vi "EPTxBasicExampleRT1.0.vi"() -> ()   [LabVIEW 2022 SP3]
uses:
  <vilib>/rvi/interface/nirviOpenFPGA/nirviOpenFPGA.xnode
  <vilib>/rvi/interface/nirviReadWriteControl/nirviReadWriteControl.xnode
  <vilib>/rvi/interface/Simulation/niFpgaSimulationCallBeginRW.vi
  <vilib>/rvi/errors/niLvFpgaAdjustHostInterfaceError.vi
  <vilib>/Powertrain Controls/Device Drivers/Engine Position Tracking/EPTx/RevA/RT/EPTx - RevA - RT.lvlib
  <vilib>/Platform/TimedLoop/XDataNode/XDataNode.xnode
  <vilib>/Platform/TimedLoop/XDataNode/nitl_modes.ctl
  <vilib>/Platform/TimedLoop/XDataNode/XDNodeRunTimeDep.lvlib
  <vilib>/Platform/TimedLoop/XDataNode/wakeup.ctl
  <vilib>/Platform/TimedLoop/XDataNode/timing_clust.ctl
  <vilib>/rvi/interface/nirviCloseFPGA/nirviCloseFPGA.xnode
  NiFpgaLv.dll
  <vilib>/Utility/error.llb/Error Cluster From Error Code.vi
  <vilib>/Powertrain Controls/Device Drivers/Engine Position Tracking/EPTx/RevA/RT/Controls/Aux Threshold.ctl
  <vilib>/Powertrain Controls/Device Drivers/Engine Position Tracking/EPTx/RevA/RT/Controls/Aux Type.ctl
  <vilib>/Powertrain Controls/Device Drivers/Engine Position Tracking/EPTx/RevA/RT/Controls/Aux Signal.ctl
  <vilib>/Powertrain Controls/Device Drivers/Engine Position Tracking/EPTx/RevA/RT/Controls/Settings - Token.ctl
  <vilib>/Powertrain Controls/Device Drivers/Engine Position Tracking/EPTx/RevA/RT/Controls/Settings - Pattern.ctl
  <vilib>/Powertrain Controls/Device Drivers/Engine Position Tracking/EPTx/RevA/RT/Controls/Direction Detection.ctl
  <vilib>/Powertrain Controls/Device Drivers/Engine Position Tracking/EPTx/RevA/RT/Controls/Settings - Tooth.ctl
  <vilib>/Powertrain Controls/Device Drivers/Engine Position Tracking/EPTx/RevA/RT/Controls/EPTxSettings.ctl
  <vilib>/Powertrain Controls/Device Drivers/Engine Position Tracking/EPTx/RevA/RT/Controls/Pattern.ctl
  <vilib>/Powertrain Controls/Device Drivers/Engine Position Tracking/EPTx/RevA/RT/Controls/EPTxPattern.ctl
  FPGA/EPTx Basic Example FPGA 1.0.vi
  <vilib>/FPGAPlugInAG/Dynamic/niLvFpga_Close_Dynamic.vi
  <vilib>/Powertrain Controls/Device Drivers/Engine Position Tracking/EPTx/RevA/RT/Controls/EPTxState.ctl
  <vilib>/Powertrain Controls/Device Drivers/Engine Position Tracking/EPTx/RevA/RT/Controls/EPTxData.ctl
  <vilib>/Powertrain Controls/Device Drivers/Engine Position Tracking/EPTx/RevA/RT/Controls/EPTxFilters.ctl
  <vilib>/Powertrain Controls/Device Drivers/Engine Position Tracking/EPTx/RevA/FPGA/Controls/EPTxDebug.ctl
  <vilib>/Powertrain Controls/Device Drivers/Engine Position Tracking/EPTx/RevA/FPGA/EPTx - RevA - FPGA.lvlib
  <vilib>/Powertrain Controls/Device Drivers/Engine Position Tracking/EPTx/RevA/RT/Controls/Pattern Config.ctl
  <vilib>/Powertrain Controls/Device Drivers/Engine Position Tracking/EPTx/RevA/RT/Controls/Simulator Config.ctl
  <vilib>/Powertrain Controls/Device Drivers/Engine Position Tracking/EPTx/RevA/RT/Controls/EPTxAAPControl.ctl
  <vilib>/userdefined/High Color/nirio_resource_hc.ctl
  <vilib>/Powertrain Controls/Device Drivers/Engine Position Tracking/EPTx/RevA/FPGA/Controls/EPTxConfig.ctl
  <vilib>/Powertrain Controls/Device Drivers/Engine Position Tracking/EPTx/RevA/FPGA/Controls/EPTxSimulatorConfig.ctl
panel:
  out "EPTxPatternSettings 2":T1
  out "EPTxSettings 2":T3 {"Pattern"."dAngle" format="%#_10g"}
  in  "Injection_DBTDC":sgl=6.0
  in  "Injection_duration[ms]":sgl=2.0
  out "EPTxSimulatorConfig":T11
  out "EPTxConfig":T12
  in  "EPTxPatternSettings":T1={"Rotations"=2, "Cylinders"=6, "Primary"=[{"Angle"=0.0, "State"=FALSE}, {"Angle"=3.0, "State"=TRUE}, {"Angle"=6.0, "State"=FALSE}, {"Angle"=9.0, "State"=TRUE}, {"Angle"=12.0, "State"=FALSE}, {"Angle"=15.0, "State"=TRUE}, {"Angle"=18.0, "State"=FALSE}, {"Angle"=21.0, "State"=TRUE}, {"Angle"=24.0, "State"=FALSE}, {"Angle"=27.0, "State"=TRUE}, {"Angle"=30.0, "State"=FALSE}, {"Angle"=33.0, "State"=TRUE}, {"Angle"=36.0, "State"=FALSE}, {"Angle"=39.0, "State"=TRUE}, {"Angle"=42.0, "State"=FALSE}, {"Angle"=45.0, "State"=TRUE}, {"Angle"=48.0, "State"=FALSE}, {"Angle"=51.0, "State"=TRUE}, {"Angle"=54.0, "State"=FALSE}, {"Angle"=57.0, "State"=TRUE}, {"Angle"=60.0, "State"=FALSE}, {"Angle"=63.0, "State"=TRUE}, {"Angle"=66.0, "State"=FALSE}, {"Angle"=69.0, "State"=TRUE}, {"Angle"=72.0, "State"=FALSE}, {"Angle"=75.0, "State"=TRUE}, {"Angle"=78.0, "State"=FALSE}, {"Angle"=81.0, "State"=TRUE}, {"Angle"=84.0, "State"=FALSE}, {"Angle"=87.0, "State"=TRUE}, {"Angle"=90.0, "State"=FALSE}, {"Angle"=93.0, "State"=TRUE}, {"Angle"=96.0, "State"=FALSE}, {"Angle"=99.0, "State"=TRUE}, {"Angle"=102.0, "State"=FALSE}, {"Angle"=105.0, "State"=TRUE}, {"Angle"=108.0, "State"=FALSE}, {"Angle"=111.0, "State"=TRUE}, {"Angle"=114.0, "State"=FALSE}, {"Angle"=117.0, "State"=TRUE}, {"Angle"=120.0, "State"=FALSE}, {"Angle"=123.0, "State"=TRUE}, {"Angle"=126.0, "State"=FALSE}, {"Angle"=129.0, "State"=TRUE}, {"Angle"=132.0, "State"=FALSE}, {"Angle"=135.0, "State"=TRUE}, {"Angle"=138.0, "State"=FALSE}, {"Angle"=141.0, "State"=TRUE}, {"Angle"=144.0, "State"=FALSE}, {"Angle"=147.0, "State"=TRUE}, {"Angle"=150.0, "State"=FALSE}, {"Angle"=153.0, "State"=TRUE}, {"Angle"=156.0, "State"=FALSE}, {"Angle"=159.0, "State"=TRUE}, {"Angle"=162.0, "State"=FALSE}, {"Angle"=165.0, "State"=TRUE}, {"Angle"=168.0, "State"=FALSE}, {"Angle"=171.0, "State"=TRUE}, {"Angle"=174.0, "State"=FALSE}, {"Angle"=177.0, "State"=TRUE}, {"Angle"=180.0, "State"=FALSE}, {"Angle"=183.0, "State"=TRUE}, {"Angle"=186.0, "State"=FALSE}, {"Angle"=189.0, "State"=TRUE}, {"Angle"=192.0, "State"=FALSE}, {"Angle"=195.0, "State"=TRUE}, {"Angle"=198.0, "State"=FALSE}, {"Angle"=201.0, "State"=TRUE}, {"Angle"=204.0, "State"=FALSE}, {"Angle"=207.0, "State"=TRUE}, {"Angle"=210.0, "State"=FALSE}, {"Angle"=213.0, "State"=TRUE}, {"Angle"=216.0, "State"=FALSE}, {"Angle"=219.0, "State"=TRUE}, {"Angle"=222.0, "State"=FALSE}, {"Angle"=225.0, "State"=TRUE}, {"Angle"=228.0, "State"=FALSE}, {"Angle"=231.0, "State"=TRUE}, {"Angle"=234.0, "State"=FALSE}, {"Angle"=237.0, "State"=TRUE}, {"Angle"=240.0, "State"=FALSE}, {"Angle"=243.0, "State"=TRUE}, {"Angle"=246.0, "State"=FALSE}, {"Angle"=249.0, "State"=TRUE}, {"Angle"=252.0, "State"=FALSE}, {"Angle"=255.0, "State"=TRUE}, {"Angle"=258.0, "State"=FALSE}, {"Angle"=261.0, "State"=TRUE}, {"Angle"=264.0, "State"=FALSE}, {"Angle"=267.0, "State"=TRUE}, {"Angle"=270.0, "State"=FALSE}, {"Angle"=273.0, "State"=TRUE}, {"Angle"=276.0, "State"=FALSE}, {"Angle"=279.0, "State"=TRUE}, {"Angle"=282.0, "State"=FALSE}, {"Angle"=285.0, "State"=TRUE}, {"Angle"=288.0, "State"=FALSE}, {"Angle"=291.0, "State"=TRUE}, {"Angle"=294.0, "State"=FALSE}, {"Angle"=297.0, "State"=TRUE}, {"Angle"=300.0, "State"=FALSE}, {"Angle"=303.0, "State"=TRUE}, {"Angle"=306.0, "State"=FALSE}, {"Angle"=309.0, "State"=TRUE}, {"Angle"=312.0, "State"=FALSE}, {"Angle"=315.0, "State"=TRUE}, {"Angle"=318.0, "State"=FALSE}, {"Angle"=321.0, "State"=TRUE}, {"Angle"=324.0, "State"=FALSE}, {"Angle"=327.0, "State"=TRUE}, {"Angle"=330.0, "State"=FALSE}, {"Angle"=333.0, "State"=TRUE}, {"Angle"=336.0, "State"=FALSE}, {"Angle"=339.0, "State"=TRUE}, {"Angle"=342.0, "State"=FALSE}, {"Angle"=345.0, "State"=TRUE}, {"Angle"=360.0, "State"=FALSE}, {"Angle"=363.0, "State"=TRUE}, {"Angle"=366.0, "State"=FALSE}, {"Angle"=369.0, "State"=TRUE}, {"Angle"=372.0, "State"=FALSE}, {"Angle"=375.0, "State"=TRUE}, {"Angle"=378.0, "State"=FALSE}, {"Angle"=381.0, "State"=TRUE}, {"Angle"=384.0, "State"=FALSE}, {"Angle"=387.0, "State"=TRUE}, {"Angle"=390.0, "State"=FALSE}, {"Angle"=393.0, "State"=TRUE}, {"Angle"=396.0, "State"=FALSE}, {"Angle"=399.0, "State"=TRUE}, {"Angle"=402.0, "State"=FALSE}, {"Angle"=405.0, "State"=TRUE}, {"Angle"=408.0, "State"=FALSE}, {"Angle"=411.0, "State"=TRUE}, {"Angle"=414.0, "State"=FALSE}, {"Angle"=417.0, "State"=TRUE}, {"Angle"=420.0, "State"=FALSE}, {"Angle"=423.0, "State"=TRUE}, {"Angle"=426.0, "State"=FALSE}, {"Angle"=429.0, "State"=TRUE}, {"Angle"=432.0, "State"=FALSE}, {"Angle"=435.0, "State"=TRUE}, {"Angle"=438.0, "State"=FALSE}, {"Angle"=441.0, "State"=TRUE}, {"Angle"=444.0, "State"=FALSE}, {"Angle"=447.0, "State"=TRUE}, {"Angle"=450.0, "State"=FALSE}, {"Angle"=453.0, "State"=TRUE}, {"Angle"=456.0, "State"=FALSE}, {"Angle"=459.0, "State"=TRUE}, {"Angle"=462.0, "State"=FALSE}, {"Angle"=465.0, "State"=TRUE}, {"Angle"=468.0, "State"=FALSE}, {"Angle"=471.0, "State"=TRUE}, {"Angle"=474.0, "State"=FALSE}, {"Angle"=477.0, "State"=TRUE}, {"Angle"=480.0, "State"=FALSE}, {"Angle"=483.0, "State"=TRUE}, {"Angle"=486.0, "State"=FALSE}, {"Angle"=489.0, "State"=TRUE}, {"Angle"=492.0, "State"=FALSE}, {"Angle"=495.0, "State"=TRUE}, {"Angle"=498.0, "State"=FALSE}, {"Angle"=501.0, "State"=TRUE}, {"Angle"=504.0, "State"=FALSE}, {"Angle"=507.0, "State"=TRUE}, {"Angle"=510.0, "State"=FALSE}, {"Angle"=513.0, "State"=TRUE}, {"Angle"=516.0, "State"=FALSE}, {"Angle"=519.0, "State"=TRUE}, {"Angle"=522.0, "State"=FALSE}, {"Angle"=525.0, "State"=TRUE}, {"Angle"=528.0, "State"=FALSE}, {"Angle"=531.0, "State"=TRUE}, {"Angle"=534.0, "State"=FALSE}, {"Angle"=537.0, "State"=TRUE}, {"Angle"=540.0, "State"=FALSE}, {"Angle"=543.0, "State"=TRUE}, {"Angle"=546.0, "State"=FALSE}, {"Angle"=549.0, "State"=TRUE}, {"Angle"=552.0, "State"=FALSE}, {"Angle"=555.0, "State"=TRUE}, {"Angle"=558.0, "State"=FALSE}, {"Angle"=561.0, "State"=TRUE}, {"Angle"=564.0, "State"=FALSE}, {"Angle"=567.0, "State"=TRUE}, {"Angle"=570.0, "State"=FALSE}, {"Angle"=573.0, "State"=TRUE}, {"Angle"=576.0, "State"=FALSE}, {"Angle"=579.0, "State"=TRUE}, {"Angle"=582.0, "State"=FALSE}, {"Angle"=585.0, "State"=TRUE}, {"Angle"=588.0, "State"=FALSE}, {"Angle"=591.0, "State"=TRUE}, {"Angle"=594.0, "State"=FALSE}, {"Angle"=597.0, "State"=TRUE}, {"Angle"=600.0, "State"=FALSE}, {"Angle"=603.0, "State"=TRUE}, {"Angle"=606.0, "State"=FALSE}, {"Angle"=609.0, "State"=TRUE}, {"Angle"=612.0, "State"=FALSE}, {"Angle"=615.0, "State"=TRUE}, {"Angle"=618.0, "State"=FALSE}, {"Angle"=621.0, "State"=TRUE}, {"Angle"=624.0, "State"=FALSE}, {"Angle"=627.0, "State"=TRUE}, {"Angle"=630.0, "State"=FALSE}, {"Angle"=633.0, "State"=TRUE}, {"Angle"=636.0, "State"=FALSE}, {"Angle"=639.0, "State"=TRUE}, {"Angle"=642.0, "State"=FALSE}, {"Angle"=645.0, "State"=TRUE}, {"Angle"=648.0, "State"=FALSE}, {"Angle"=651.0, "State"=TRUE}, {"Angle"=654.0, "State"=FALSE}, {"Angle"=657.0, "State"=TRUE}, {"Angle"=660.0, "State"=FALSE}, {"Angle"=663.0, "State"=TRUE}, {"Angle"=666.0, "State"=FALSE}, {"Angle"=669.0, "State"=TRUE}, {"Angle"=672.0, "State"=FALSE}, {"Angle"=675.0, "State"=TRUE}, {"Angle"=678.0, "State"=FALSE}, {"Angle"=681.0, "State"=TRUE}, {"Angle"=684.0, "State"=FALSE}, {"Angle"=687.0, "State"=TRUE}, {"Angle"=690.0, "State"=FALSE}, {"Angle"=693.0, "State"=TRUE}, {"Angle"=696.0, "State"=FALSE}, {"Angle"=699.0, "State"=TRUE}, {"Angle"=702.0, "State"=FALSE}, {"Angle"=705.0, "State"=TRUE}], "Aux 1"=[{"Angle"=12.0, "State"=TRUE}, {"Angle"=24.0, "State"=FALSE}, {"Angle"=48.0, "State"=TRUE}, {"Angle"=60.0, "State"=FALSE}, {"Angle"=132.0, "State"=TRUE}, {"Angle"=144.0, "State"=FALSE}, {"Angle"=198.0, "State"=TRUE}, {"Angle"=252.0, "State"=TRUE}, {"Angle"=264.0, "State"=FALSE}, {"Angle"=318.0, "State"=TRUE}, {"Angle"=372.0, "State"=TRUE}, {"Angle"=384.0, "State"=FALSE}, {"Angle"=438.0, "State"=TRUE}, {"Angle"=492.0, "State"=TRUE}, {"Angle"=504.0, "State"=FALSE}, {"Angle"=558.0, "State"=TRUE}, {"Angle"=612.0, "State"=TRUE}, {"Angle"=624.0, "State"=FALSE}, {"Angle"=678.0, "State"=TRUE}], "Aux 2"=[{"Angle"=12.0, "State"=TRUE}, {"Angle"=24.0, "State"=FALSE}, {"Angle"=48.0, "State"=TRUE}, {"Angle"=60.0, "State"=FALSE}, {"Angle"=132.0, "State"=TRUE}, {"Angle"=144.0, "State"=FALSE}, {"Angle"=198.0, "State"=TRUE}, {"Angle"=252.0, "State"=TRUE}, {"Angle"=264.0, "State"=FALSE}, {"Angle"=318.0, "State"=TRUE}, {"Angle"=372.0, "State"=TRUE}, {"Angle"=384.0, "State"=FALSE}, {"Angle"=438.0, "State"=TRUE}, {"Angle"=492.0, "State"=TRUE}, {"Angle"=504.0, "State"=FALSE}, {"Angle"=558.0, "State"=TRUE}, {"Angle"=612.0, "State"=TRUE}, {"Angle"=624.0, "State"=FALSE}, {"Angle"=678.0, "State"=TRUE}], "Aux 3"=[], "Aux 4"=[]}
  in  "load_备用":bool
  out "EPTxSettings":T3 {"Pattern"."dAngle" format="%#_10g"}
  in  "EPTxAAPControl_6str":T13={"Enable"=FALSE, "Rising [DBTDC]"=12.0, "Falling [DBTDC]"=-12.0}
  in  "EPTxAAPControl_5str":T13={"Enable"=FALSE, "Rising [DBTDC]"=12.0, "Falling [DBTDC]"=-12.0}
  in  "EPTxAAPControl_4str":T13={"Enable"=FALSE, "Rising [DBTDC]"=12.0, "Falling [DBTDC]"=-12.0}
  in  "EPTxAAPControl_3str":T13={"Enable"=FALSE, "Rising [DBTDC]"=12.0, "Falling [DBTDC]"=-12.0}
  in  "EPTxAAPControl_2str":T13={"Enable"=FALSE, "Rising [DBTDC]"=12.0, "Falling [DBTDC]"=-12.0}
  out "Loop":u32
  in  "资源名称":T14="PXI1Slot7" caption="RIO设备"
  out "Config Loading":bool
  in  "EPTxAAPControl_1str":T13={"Enable"=FALSE, "Rising [DBTDC]"=12.0, "Falling [DBTDC]"=-12.0}
  out "Pattern Loading":bool
  in  "SimulatorConfig":T15={"Sim Speed [RPM]"=1000.0, "Ramp Rate [RPM/s]"=50.0, "Rotations"=2, "Pause"=FALSE, "Pause Angle [CAD]"=0.0, "Max Offset [RPM]"=0.0, "Cylinders"=6}
  out "Sim Loading":bool
  in  "PatternConfig":T16 {"Max Rate [Hz]" format="%#_3p"}
  out "error out":errorcluster
  out "RT Loop Iteration Duration":i64 caption="[ms]"
  out "EPTxDebug":T17={"Sync"=TRUE, "CycleCount"=146.0, "StartCAD"=0.0, "EndCAD"=123.3046875}
  in  "History [CAD]":u8=63
  in  "EPTxFilters":T18={"Primary [s]"=5e-06, "Aux 1 [s]"=5e-06, "Aux 2 [s]"=0.0, "Aux 3 [s]"=0.0, "Aux 4 [s]"=0.0} {"Aux 4 [s]" format="%#_6p"; "Aux 3 [s]" format="%#_6p"; "Aux 2 [s]" format="%#_6p"; "Aux 1 [s]" format="%#_6p"; "Primary [s]" format="%#_6p"}
  in  "Stall Speed [RPM]":sgl=200.0
  in  "Configuration Filename":string="YC-6kcfg.EPTx"
  in  "Pattern Filename":string="YC-6kcfg.EPTxP"
  in  "Load":bool
  out "EPTxData":T19={"Sync"=TRUE, "CurrentCAD"=122.91406, "Speed [RPM]"=999.75, "Config"=FALSE, "Rcvg Primary"=TRUE, "Stall"=FALSE, "Overflow"=FALSE, "Ratio Error"=FALSE, "Pattern Error"=FALSE, "Aux Warning"=FALSE, "Watchdog Error"=FALSE}
  in  "EPTxState":T20={"Sync Enable"=TRUE, "Clear Errors"=FALSE, "Sim Enable"=FALSE, "Sim Speed [RPM]"=1000.0}
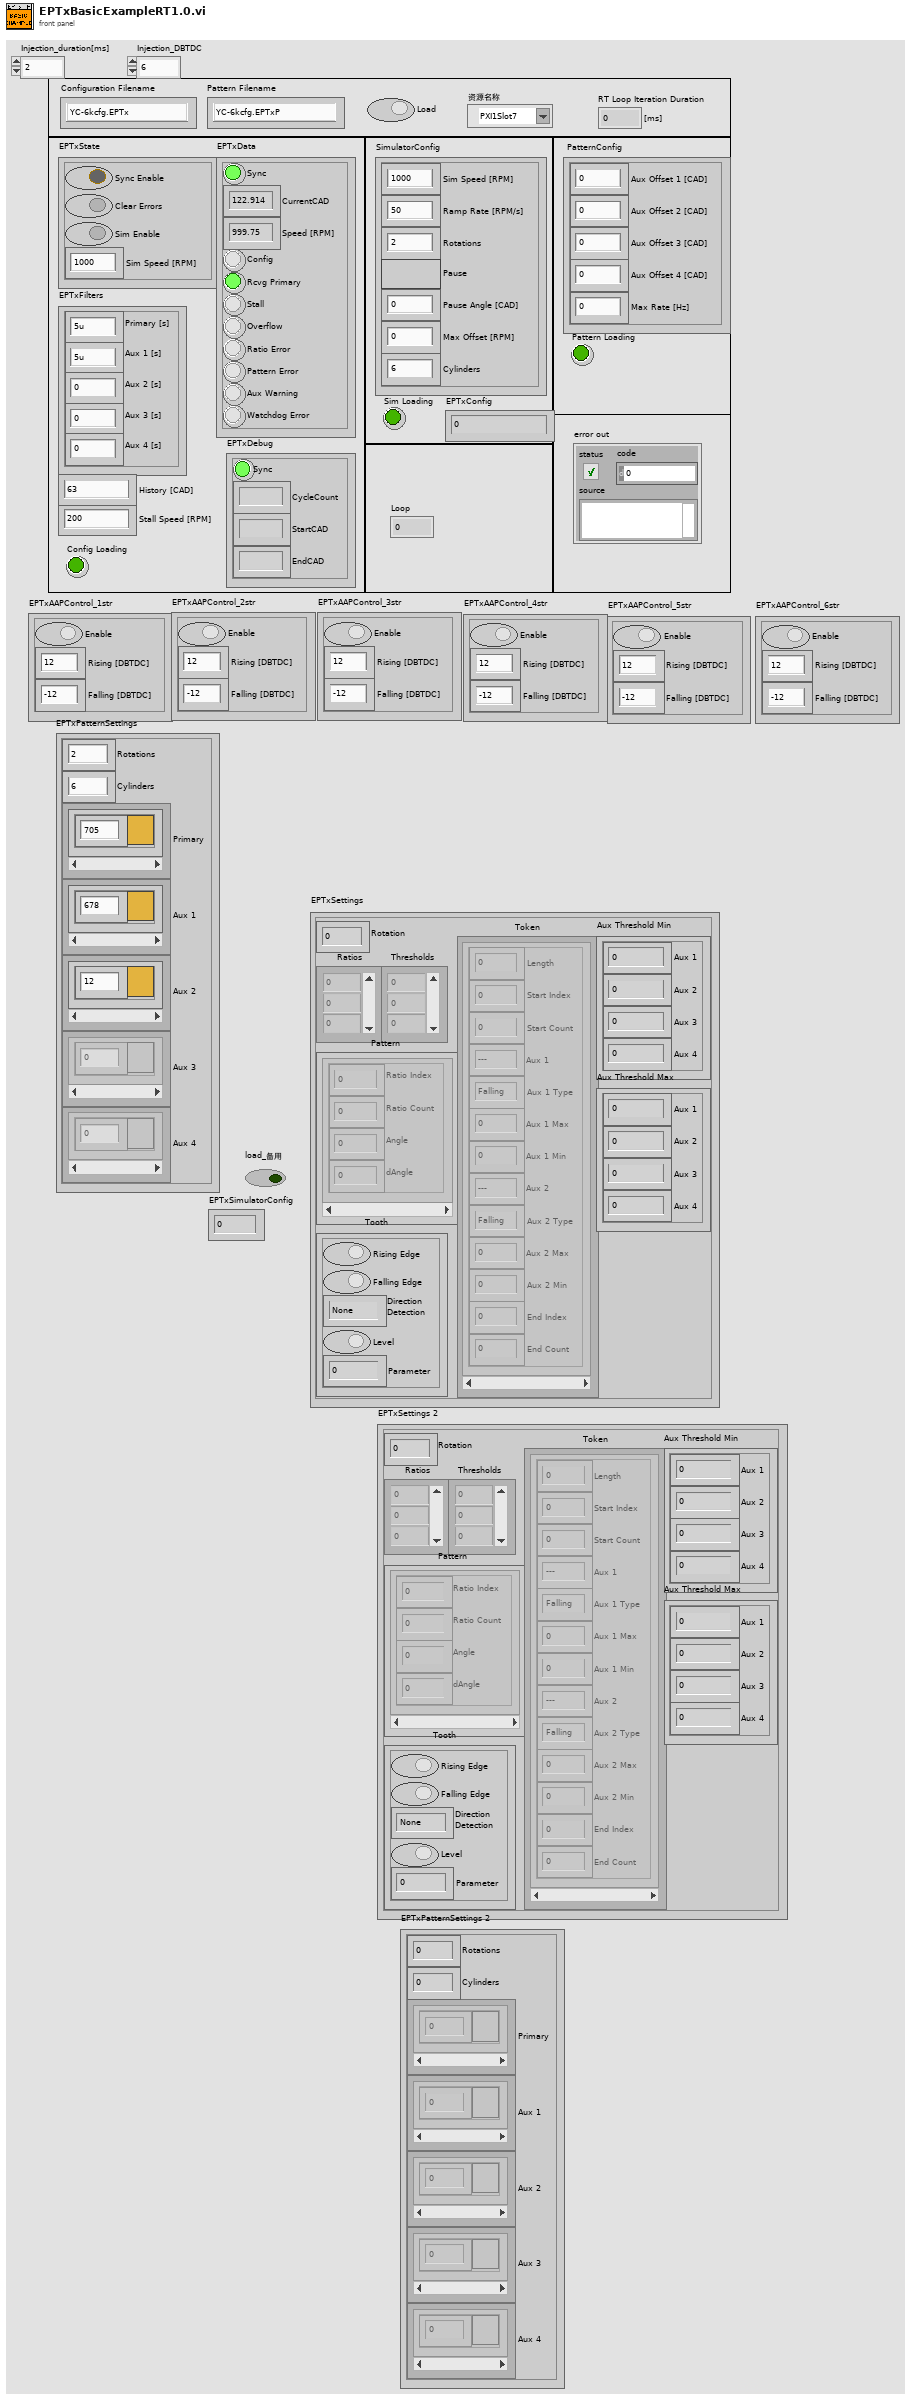
[diagram p1: front panel]
types:
  T1 = typedef "EPTx - RevA - RT.lvlib/EPTxPattern.ctl" = cluster{"Rotations":u8, "Cylinders":u8, "Primary":T2[], "Aux 1":T2[], "Aux 2":T2[], "Aux 3":T2[], "Aux 4":T2[]}
  T2 = typedef "EPTx - RevA - RT.lvlib/Pattern.ctl" = cluster{"Angle":sgl, "State":bool}
  T3 = typedef "EPTx - RevA - RT.lvlib/EPTxSettings.ctl" = cluster{"Rotation":u8, "Ratios":sgl[], "Thresholds":sgl[], "Tooth":T4, "Pattern":T6[], "Token":T7[], "Aux Threshold Min":T10, "Aux Threshold Max":T10}
  T4 = typedef "EPTx - RevA - RT.lvlib/Settings - Tooth.ctl" = cluster{"Rising Edge":bool, "Falling Edge":bool, "Direction\nDetection":T5, "Level":bool, "Parameter":sgl}
  T5 = typedef "EPTx - RevA - RT.lvlib/Direction Detection.ctl" = enum16{"None", "Aux Signal", "Length"}
  T6 = typedef "EPTx - RevA - RT.lvlib/Settings - Pattern.ctl" = cluster{"Ratio Index":u8, "Ratio Count":u16, "Angle":sgl, "dAngle":sgl}
  T7 = typedef "EPTx - RevA - RT.lvlib/Settings - Token.ctl" = cluster{"Length":u16, "Start Index":u8, "Start Count":u16, "Aux 1":T8, "Aux 1 Type":T9, "Aux 1 Max":u16, "Aux 1 Min":u16, "Aux 2":T8, "Aux 2 Type":T9, "Aux 2 Max":u16, "Aux 2 Min":u16, "End Index":u8, "End Count":u16}
  T8 = typedef "EPTx - RevA - RT.lvlib/Aux Signal.ctl" = enum8{"---", "Aux 1", "Aux 2", "Aux 3", "Aux 4"}
  T9 = typedef "EPTx - RevA - RT.lvlib/Aux Type.ctl" = enum8{"Falling", "Rising", "Low", "High", "Ratio"}
  T10 = typedef "EPTx - RevA - RT.lvlib/Aux Threshold.ctl" = cluster{"Aux 1":sgl, "Aux 2":sgl, "Aux 3":sgl, "Aux 4":sgl}
  T11 = typedef "EPTx - RevA - FPGA.lvlib/EPTxSimulatorConfig.ctl" = u32
  T12 = typedef "EPTx - RevA - FPGA.lvlib/EPTxConfig.ctl" = u64
  T13 = typedef "EPTx - RevA - RT.lvlib/EPTxAAPControl.ctl" = cluster{"Enable":bool, "Rising [DBTDC]":sgl, "Falling [DBTDC]":sgl}
  T14 = typedef "nirio_resource_hc.ctl" = tag
  T15 = typedef "EPTx - RevA - RT.lvlib/Simulator Config.ctl" = cluster{"Sim Speed [RPM]":sgl, "Ramp Rate [RPM/s]":sgl, "Rotations":u8, "Pause":bool, "Pause Angle [CAD]":sgl, "Max Offset [RPM]":sgl, "Cylinders":u8}
  T16 = typedef "EPTx - RevA - RT.lvlib/Pattern Config.ctl" = cluster{"Aux Offset 1 [CAD]":sgl, "Aux Offset 2 [CAD]":sgl, "Aux Offset 3 [CAD]":sgl, "Aux Offset 4 [CAD]":sgl, "Max Rate [Hz]":sgl}
  T17 = typedef "EPTx - RevA - FPGA.lvlib/EPTxDebug.ctl" = cluster{"Sync":bool, "CycleCount":fxp<+,8,8>, "StartCAD":fxp<+,18,11>, "EndCAD":fxp<+,18,11>}
  T18 = typedef "EPTx - RevA - RT.lvlib/EPTxFilters.ctl" = cluster{"Primary [s]":sgl, "Aux 1 [s]":sgl, "Aux 2 [s]":sgl, "Aux 3 [s]":sgl, "Aux 4 [s]":sgl}
  T19 = typedef "EPTx - RevA - RT.lvlib/EPTxData.ctl" = cluster{"Sync":bool, "CurrentCAD":sgl, "Speed [RPM]":sgl, "Config":bool, "Rcvg Primary":bool, "Stall":bool, "Overflow":bool, "Ratio Error":bool, "Pattern Error":bool, "Aux Warning":bool, "Watchdog Error":bool}
  T20 = typedef "EPTx - RevA - RT.lvlib/EPTxState.ctl" = cluster{"Sync Enable":bool, "Clear Errors":bool, "Sim Enable":bool, "Sim Speed [RPM]":sgl}
  T21 = typedef "XDNodeRunTimeDep.lvlib/timing_clust.ctl" = cluster{"Expected End [f-1]":u64, "Actual End [f-1]":u64, "Finished Late? [f-1]":bool, "Expected End [i-1]":u64, "Actual End [i-1]":u64, "Finished Late? [i-1]":bool, "Expected Start [i]":u64, "Actual Start [i]":u64, "Expected Start [f]":u64, "Actual Start [f]":u64, "Source Name":string, "Structure Name":string, "Period":i64, "Deadline":i64, "Offset":i64, "Start":i64, "Priority":i32, "Timeout":i32, "Mode":T22, "Wakeup Reason":T23, "Error":errorcluster, "Source Type":string, "Secondary Source Type":string, "Global End Time":u64, "Global Start Time":u64, "Frame Duration":u64, "Iteration Duration":u64, "Assigned CPU":i32, "I/O Scan Engine Mode":u32}
  T22 = typedef "XDNodeRunTimeDep.lvlib/nitl_modes.ctl" = enum32{"No Change", "Process missed periods, maintain original phase", "Discard missed periods, maintain original phase", "Process missed periods, ignore original phase", "Discard missed periods, ignore original phase"}
  T23 = typedef "XDNodeRunTimeDep.lvlib/wakeup.ctl" = enum32{"Normal", "Aborted", "Asynchronous wakeup", "Timing source error", "Timed loop error", "Timeout"}
  T24 = cluster{"Cylinder6_H_R [CAD]":fxp<+,18,11>, "Cylinder6_H_F [CAD]":fxp<+,18,11>}
  T25 = cluster{"Cylinder5_H_R [CAD]":fxp<+,18,11>, "Cylinder5_H_F [CAD]":fxp<+,18,11>}
  T26 = cluster{"Cylinder4_H_R [CAD]":fxp<+,18,11>, "Cylinder4_H_F [CAD]":fxp<+,18,11>}
  T27 = cluster{"Cylinder3_H_R [CAD]":fxp<+,18,11>, "Cylinder3_H_F [CAD]":fxp<+,18,11>}
  T28 = cluster{"Cylinder2_H_R [CAD]":fxp<+,18,11>, "Cylinder2_H_F [CAD]":fxp<+,18,11>}
  T29 = cluster{"Cylinder1_H_R [CAD]":fxp<+,18,11>, "Cylinder1_H_F [CAD]":fxp<+,18,11>}
  T30 = cluster{"Sync":bool, "CurrentCAD":fxp<+,18,11>, "MaxCAD":fxp<+,11,11>, "HistoryCAD":fxp<+,11,11>, "CADRate":fxp<+,22,8>, "AvgSpeed":fxp<+,17,15>, "Config":bool, "Rcvg Primary":bool, "Stall":bool, "Overflow":bool, "Ratio Error":bool, "Pattern Error":bool, "Aux Warning":bool, "Watchdog Error":bool}
  T31 = typedef "EPTx - RevA - FPGA.lvlib/EPTxControl.ctl" = cluster{"Sync Enable":bool, "Clear Errors":bool, "Sim Enable":bool, "Sim Rate":fxp<+,24,6>, "Watchdog":bool}
  T32 = typedef "EPTx - RevA - FPGA.lvlib/EPTxPatternConfig.ctl" = cluster{"Address":fxp<+,14,14>, "Pattern":T33}
  T33 = typedef "EPTx - RevA - FPGA.lvlib/Patterns.ctl" = cluster{"Primary":fxp<+,19,12>, "Primary State":bool, "Aux 1":fxp<+,19,12>, "Aux 1 State":bool, "Aux 2":fxp<+,19,12>, "Aux 2 State":bool, "Aux 3":fxp<+,19,12>, "Aux 3 State":bool, "Aux 4":fxp<+,19,12>, "Aux 4 State":bool}
  T34 = cluster{"Sync":bool, "CycleCount":fxp<+,8,8>, "StartCAD":fxp<+,18,11>, "EndCAD":fxp<+,18,11>}
  T35 = typedef "EPTx - RevA - FPGA.lvlib/EPTxAAPControl.ctl" = cluster{"Enable":bool, "RisingCAD":fxp<+,18,11>, "FallingCAD":fxp<+,18,11>}
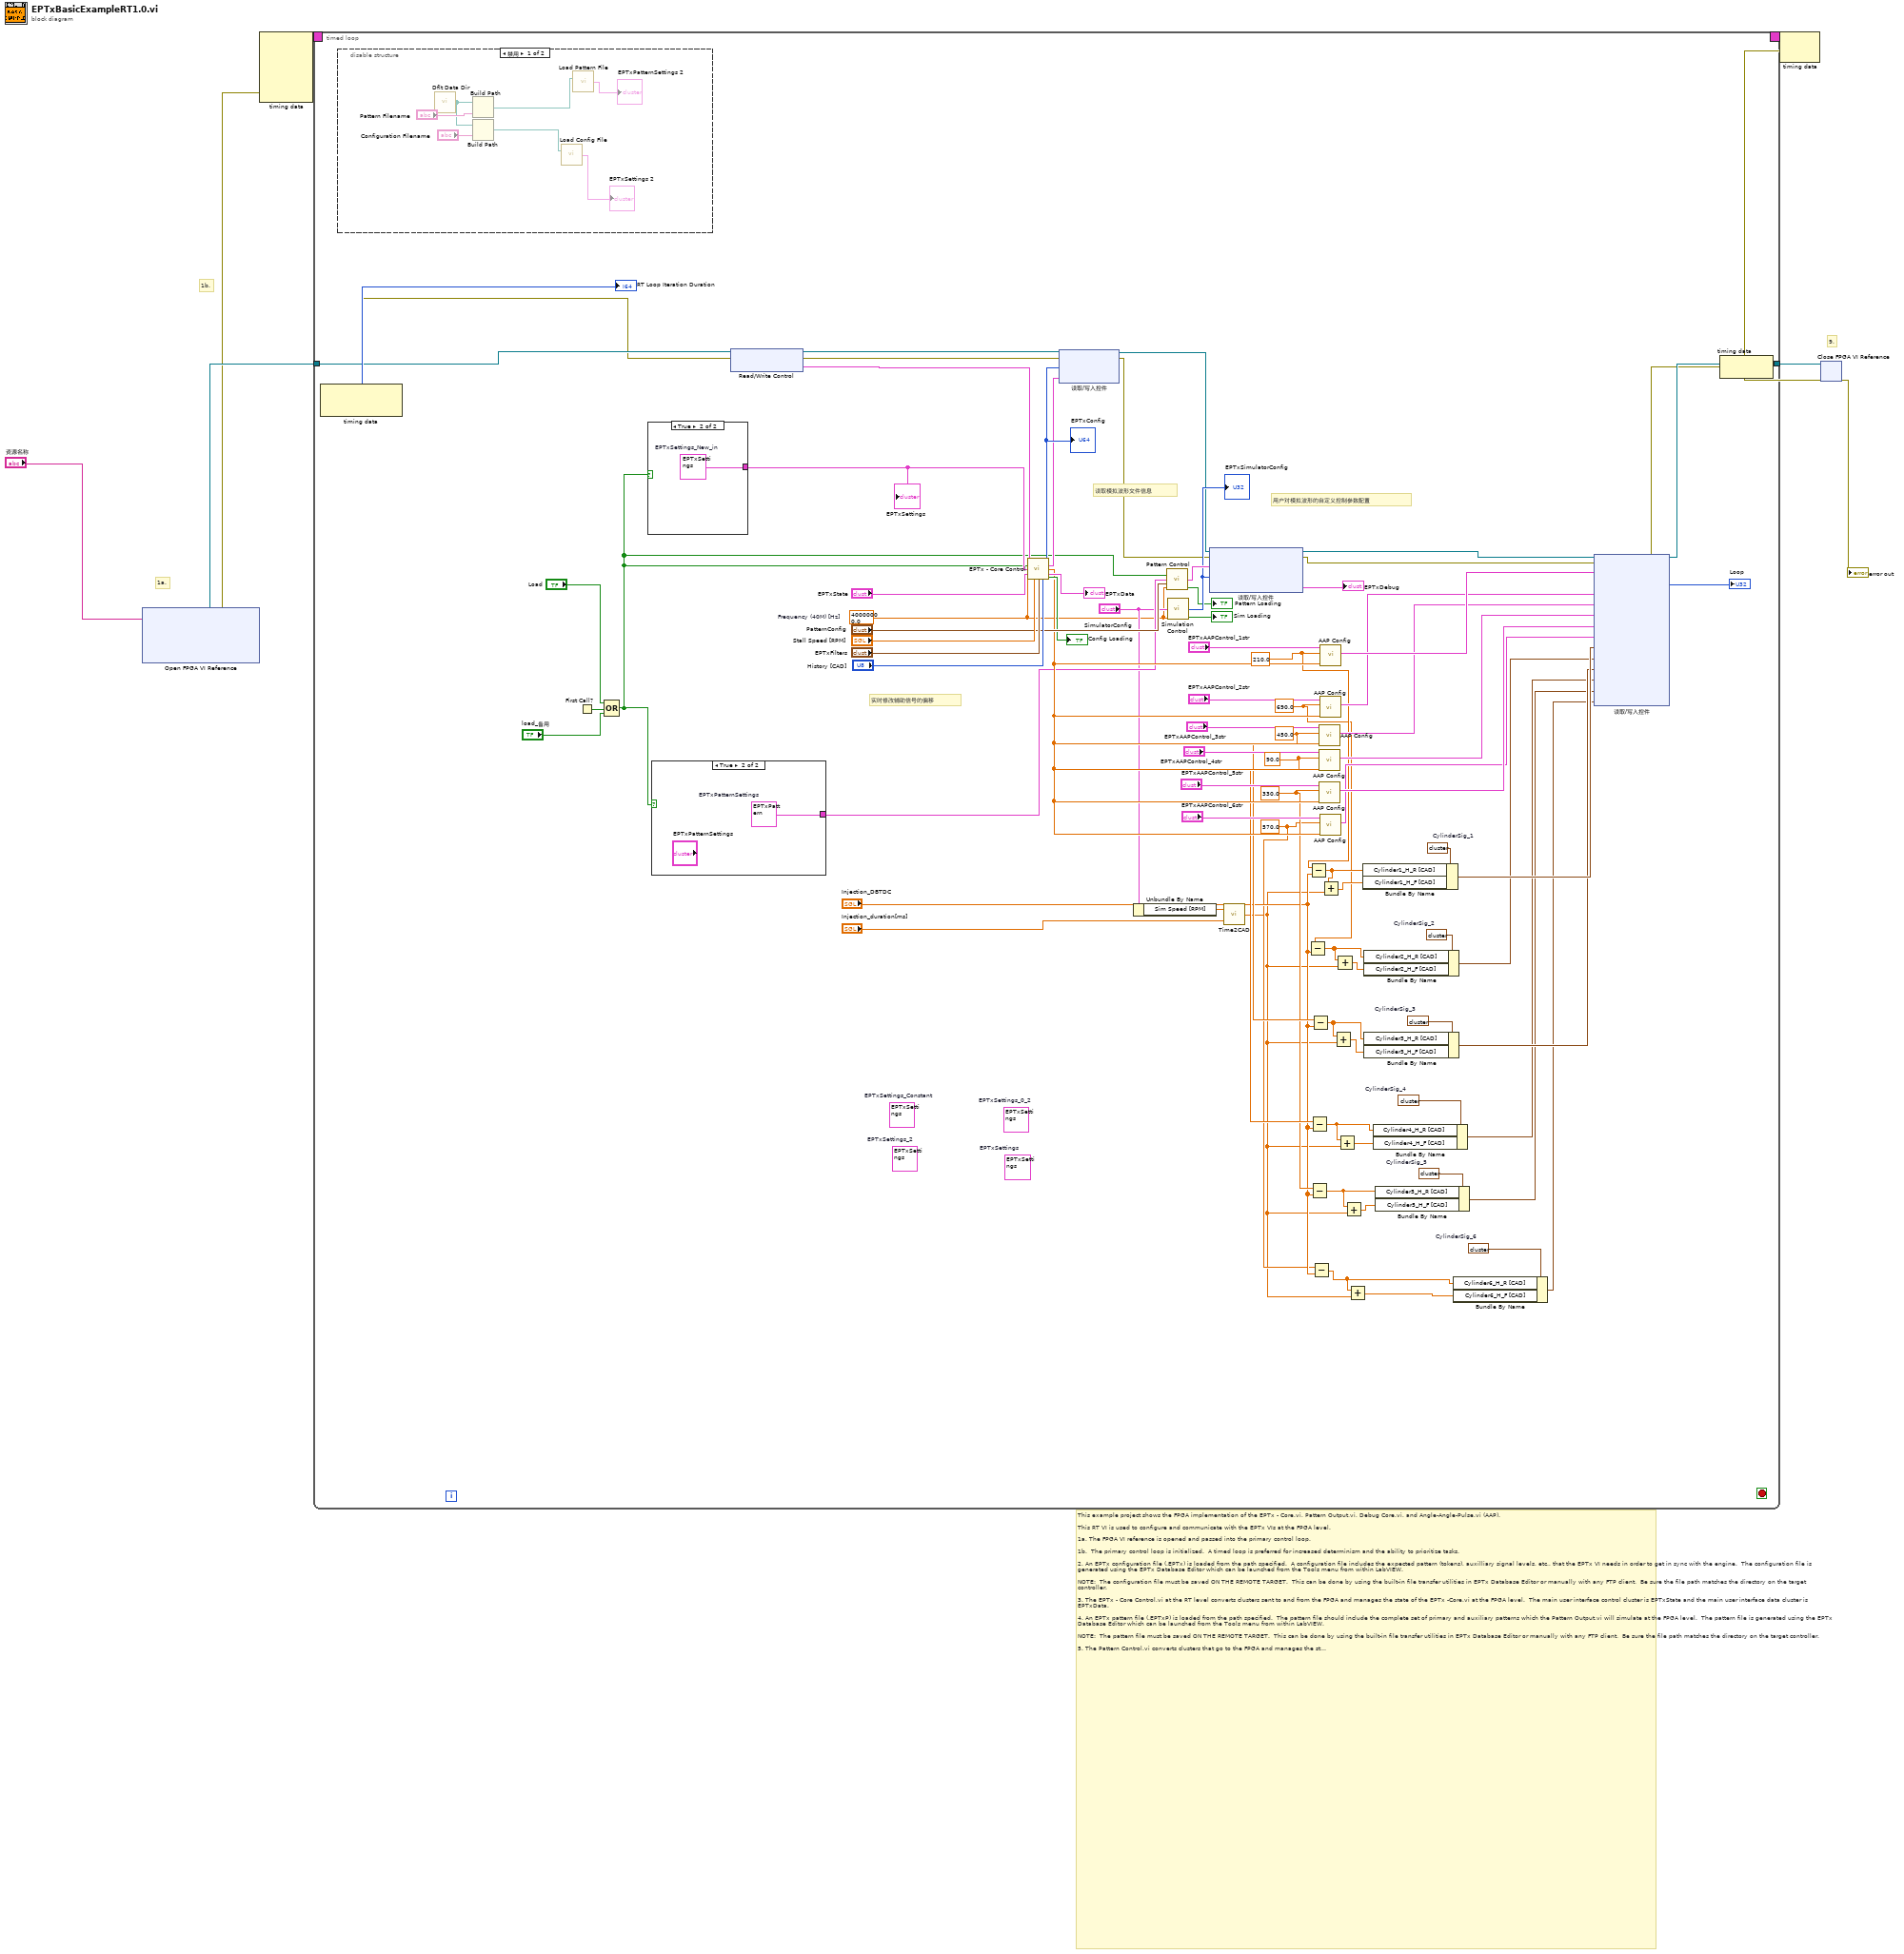
[diagram p0: block diagram]
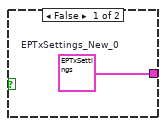
[diagram p3: hidden frame]
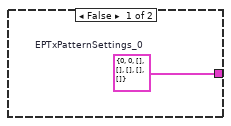
[diagram p4: hidden frame]
diagram:
  # "9."
  # "1b."
  # "1a."
  # "This example project shows the FPGA implementation of the EPTx - Core.vi, Pattern Output.vi, Debug Core.vi, and Angle-Angle-Pulse.vi (AAP).\n\nThis RT VI is used to configure and communicate with the EPTx VIs at the FPGA level.\n\n1a. The FPGA VI reference is opened and passed into the primary control loop.\n\n1b.  The primary control loop is initialized.  A timed loop is preferred for increased determinism and the ability to prioritize tasks.\n\n2. An EPTx configuration file (.EPTx) is loaded from the path specified.  A configuration file includes the expected pattern (tokens), auxilliary signal levels, etc., that the EPTx VI needs in order to get in sync with the engine.  The configuration file is generated using the EPTx Database Editor which can be launched from the Tools menu from within LabVIEW.\n\nNOTE:  The configuration file must be saved ON THE REMOTE TARGET.  This can be done by using the built-in file transfer utilities in EPTx Database Editor or manually with any FTP client.  Be sure the file path matches the directory on the target controller.\n\n3. The EPTx - Core Control.vi at the RT level converts clusters sent to and from the FPGA and manages the state of the EPTx -Core.vi at the FPGA level.  The main user interface control cluster is EPTxState and the main user interface data cluster is EPTxData.\n\n4. An EPTx pattern file (.EPTxP) is loaded from the path specified.  The pattern file should include the complete set of primary and auxiliary patterns which the Pattern Output.vi will simulate at the FPGA level.  The pattern file is generated using the EPTx Database Editor which can be launched from the Tools menu from within LabVIEW.\n\nNOTE:  The pattern file must be saved ON THE REMOTE TARGET.  This can be done by using the built-in file transfer utilities in EPTx Database Editor or manually with any FTP client.  Be sure the file path matches the directory on the target controller.\n\n5. The Pattern Control.vi converts clusters that go to the FPGA and manages the state of the Pattern Output.vi at the FPGA level.  The main user interface control cluster is Pattern Config.  The 'Loading' output indicates the RT VI is busy sending information to the FPGA.\n\n6.  The Simulation Control.vi converts clusters that go to the FPGA and manages the state of the Simulator.vi at the FPGA level.  The main user interface control cluster is Simulator Config.  The 'Loading' output indicates the RT VI is busy sending information to the FPGA.\n\n7. The EPTxDebug cluster reports data from the Debug Core.vi at the FPGA level which includes information that may help the user debug issues with achieving or losing sync.\n\n8. Controls to EPTx Extra blocks.  In this example, an Angle-Angle-Pulse (AAP) VI is used to generate an engine-synchronous boolean pulse.\n\n9. Close the FPGA VI reference."
  n1 = xnode "Open FPGA VI Reference"("resource name"="资源名称") -> ("FPGA VI Reference Out"=w8:refnum<k20>, "error out"=w3:errorcluster)  [unwired: 1 in]
  n2 = node-c288(w3) -> (w7:T21)  [unwired: 4 in]
  n3 = timed-loop {
    tunnel: w8 -> [w53]
    timing: w7 -> [_]
    timing-out: [_] -> w6
    tunnel: [w80] -> w5
    stop <- _ stop-if-true
    w16 = T24 {"Cylinder6_H_R [CAD]"=0.0, "Cylinder6_H_F [CAD]"=0.0}  # CylinderSig_6
    w24 = T25 {"Cylinder5_H_R [CAD]"=324.0, "Cylinder5_H_F [CAD]"=330.0}  # CylinderSig_5
    w29 = T26 {"Cylinder4_H_R [CAD]"=90.0, "Cylinder4_H_F [CAD]"=100.0}  # CylinderSig_4
    w35 = T27 {"Cylinder3_H_R [CAD]"=444.0, "Cylinder3_H_F [CAD]"=450.0}  # CylinderSig_3
    w38 = T28 {"Cylinder2_H_R [CAD]"=684.0, "Cylinder2_H_F [CAD]"=690.0}  # CylinderSig_2
    w42 = T29 {"Cylinder1_H_R [CAD]"=204.0, "Cylinder1_H_F [CAD]"=210.0}  # CylinderSig_1
    (unwired) T3 {"Rotation"=2, "Ratios"=[0.33333334, 1.0, 3.0], "Thresholds"=[0.16666667, 0.6666667, 0.6666667, 2.0, 2.0, 4.0, 999.0], "Tooth"={"Rising Edge"=TRUE, "Falling Edge"=FALSE, "Direction\nDetection"=enum."None", "Level"=FALSE, "Parameter"=0.0}, "Pattern"=[{"Ratio Index"=0, "Ratio Count"=1, "Angle"=0.0, "dAngle"=6.0}, {"Ratio Index"=1, "Ratio Count"=56, "Angle"=6.0, "dAngle"=6.0}, {"Ratio Index"=2, "Ratio Count"=1, "Angle"=342.0, "dAngle"=18.0}, {"Ratio Index"=0, "Ratio Count"=1, "Angle"=360.0, "dAngle"=6.0}, {"Ratio Index"=1, "Ratio Count"=56, "Angle"=366.0, "dAngle"=6.0}, {"Ratio Index"=2, "Ratio Count"=1, "Angle"=702.0, "dAngle"=18.0}], "Token"=[{"Length"=1, "Start Index"=5, "Start Count"=0, "Aux 1"=enum."---", "Aux 1 Type"=enum."Falling", "Aux 1 Max"=0, "Aux 1 Min"=0, "Aux 2"=enum."Aux 2", "Aux 2 Type"=enum."Ratio", "Aux 2 Max"=73, "Aux 2 Min"=73, "End Index"=0, "End Count"=0}], "Aux Threshold Min"={"Aux 1"=2.3333333, "Aux 2"=1.4285715, "Aux 3"=0.0, "Aux 4"=0.0}, "Aux Threshold Max"={"Aux 1"=2.3333333, "Aux 2"=1.4285715, "Aux 3"=999.0, "Aux 4"=999.0}}  # EPTxSettings
    (unwired) T3 {"Rotation"=0, "Ratios"=[], "Thresholds"=[], "Tooth"={"Rising Edge"=FALSE, "Falling Edge"=FALSE, "Direction\nDetection"=enum."None", "Level"=FALSE, "Parameter"=0.0}, "Pattern"=[], "Token"=[], "Aux Threshold Min"={"Aux 1"=0.0, "Aux 2"=0.0, "Aux 3"=0.0, "Aux 4"=0.0}, "Aux Threshold Max"={"Aux 1"=0.0, "Aux 2"=0.0, "Aux 3"=0.0, "Aux 4"=0.0}}  # EPTxSettings_0_2
    (unwired) T3 {"Rotation"=0, "Ratios"=[], "Thresholds"=[], "Tooth"={"Rising Edge"=FALSE, "Falling Edge"=FALSE, "Direction\nDetection"=enum."None", "Level"=FALSE, "Parameter"=0.0}, "Pattern"=[], "Token"=[], "Aux Threshold Min"={"Aux 1"=0.0, "Aux 2"=0.0, "Aux 3"=0.0, "Aux 4"=0.0}, "Aux Threshold Max"={"Aux 1"=0.0, "Aux 2"=0.0, "Aux 3"=0.0, "Aux 4"=0.0}}  # EPTxSettings_Constant
    (unwired) T3 {"Rotation"=2, "Ratios"=[0.33333334, 1.0, 3.0], "Thresholds"=[0.16666667, 0.6666667, 0.6666667, 2.0, 2.0, 4.0, 999.0], "Tooth"={"Rising Edge"=TRUE, "Falling Edge"=FALSE, "Direction\nDetection"=enum."None", "Level"=FALSE, "Parameter"=0.0}, "Pattern"=[{"Ratio Index"=0, "Ratio Count"=1, "Angle"=0.0, "dAngle"=6.0}, {"Ratio Index"=1, "Ratio Count"=56, "Angle"=6.0, "dAngle"=6.0}, {"Ratio Index"=2, "Ratio Count"=1, "Angle"=342.0, "dAngle"=18.0}, {"Ratio Index"=0, "Ratio Count"=1, "Angle"=360.0, "dAngle"=6.0}, {"Ratio Index"=1, "Ratio Count"=56, "Angle"=366.0, "dAngle"=6.0}, {"Ratio Index"=2, "Ratio Count"=1, "Angle"=702.0, "dAngle"=18.0}], "Token"=[{"Length"=1, "Start Index"=5, "Start Count"=0, "Aux 1"=enum."---", "Aux 1 Type"=enum."Falling", "Aux 1 Max"=0, "Aux 1 Min"=0, "Aux 2"=enum."Aux 2", "Aux 2 Type"=enum."Ratio", "Aux 2 Max"=73, "Aux 2 Min"=73, "End Index"=0, "End Count"=0}], "Aux Threshold Min"={"Aux 1"=2.3333333, "Aux 2"=1.4285715, "Aux 3"=0.0, "Aux 4"=0.0}, "Aux Threshold Max"={"Aux 1"=2.3333333, "Aux 2"=1.4285715, "Aux 3"=999.0, "Aux 4"=999.0}}  # EPTxSettings_2
    w18 = sgl 570.0 ("Cylinder TDC [Absolute CAD]")
    w22 = sgl 330.0 ("Cylinder TDC [Absolute CAD]")
    w27 = sgl 90.0 ("Cylinder TDC [Absolute CAD]")
    w33 = sgl 450.0 ("Cylinder TDC [Absolute CAD]")
    w37 = sgl 690.0 ("Cylinder TDC [Absolute CAD]")
    w43 = sgl 210.0 ("Cylinder TDC [Absolute CAD]")
    w11 = sgl 40000000.0  # Frequency (40M) [Hz]
    # "实时修改辅助信号的偏移"
    # "读取模拟波形文件信息"
    # "用户对模拟波形的自定义控制参数配置"
    n4 = node-c288() -> (→"RT Loop Iteration Duration":i64, w52:errorcluster)  [unwired: 1 in]
    n5 = disable-structure shown="禁用" {
      frame Disabled {
        n6 = call <vilib>:"Dflt Data Dir.vi"() -> ("App:Default Data Directory"=w95:path)
        n7 = Build Path(base path=w95, name or relative path="Pattern Filename") -> (appended path=w92:path)
        n8 = Build Path(base path=w95, name or relative path="Configuration Filename") -> (appended path=w94:path)
        n9 = call <vilib>:"Load Config File.vi"("Configuration Path"=w94) -> ("EPTxSettings"=→"EPTxSettings 2":T3)  [unwired: 13 in, 1 out]
        n10 = call <vilib>:"Load Pattern File.vi"("Pattern Path"=w92) -> ("EPTxPatternSettings"=→"EPTxPatternSettings 2":T1)  [unwired: 13 in, 1 out]
      }
      frame Enabled {
      }
    }
    n11 = First Call?() -> (First Call?: T/F=w57:bool)
    n12 = Compound Arithmetic op=OR ("复合运算")("Load", w57, "load_备用") -> (w9:bool)
    n13 = case shown="True" w9 {
      tunnel: [w98 w99] -> w46
      frame False {
        w98 = T3 {"Rotation"=0, "Ratios"=[], "Thresholds"=[], "Tooth"={"Rising Edge"=FALSE, "Falling Edge"=FALSE, "Direction\nDetection"=enum."None", "Level"=FALSE, "Parameter"=0.0}, "Pattern"=[], "Token"=[], "Aux Threshold Min"={"Aux 1"=0.0, "Aux 2"=0.0, "Aux 3"=0.0, "Aux 4"=0.0}, "Aux Threshold Max"={"Aux 1"=0.0, "Aux 2"=0.0, "Aux 3"=0.0, "Aux 4"=0.0}}  # EPTxSettings_New_0
      }
      frame True {
        w99 = T3 {"Rotation"=2, "Ratios"=[0.33333334, 1.0, 3.0], "Thresholds"=[0.16666667, 0.6666667, 0.6666667, 2.0, 2.0, 4.0, 999.0], "Tooth"={"Rising Edge"=TRUE, "Falling Edge"=FALSE, "Direction\nDetection"=enum."None", "Level"=FALSE, "Parameter"=0.0}, "Pattern"=[{"Ratio Index"=0, "Ratio Count"=1, "Angle"=0.0, "dAngle"=6.0}, {"Ratio Index"=1, "Ratio Count"=56, "Angle"=6.0, "dAngle"=6.0}, {"Ratio Index"=2, "Ratio Count"=1, "Angle"=342.0, "dAngle"=18.0}, {"Ratio Index"=0, "Ratio Count"=1, "Angle"=360.0, "dAngle"=6.0}, {"Ratio Index"=1, "Ratio Count"=56, "Angle"=366.0, "dAngle"=6.0}, {"Ratio Index"=2, "Ratio Count"=1, "Angle"=702.0, "dAngle"=18.0}], "Token"=[{"Length"=1, "Start Index"=5, "Start Count"=0, "Aux 1"=enum."---", "Aux 1 Type"=enum."Falling", "Aux 1 Max"=0, "Aux 1 Min"=0, "Aux 2"=enum."Aux 2", "Aux 2 Type"=enum."Ratio", "Aux 2 Max"=73, "Aux 2 Min"=73, "End Index"=0, "End Count"=0}], "Aux Threshold Min"={"Aux 1"=1.8809524, "Aux 2"=1.2142857, "Aux 3"=0.0, "Aux 4"=0.0}, "Aux Threshold Max"={"Aux 1"=2.7857144, "Aux 2"=1.8809524, "Aux 3"=999.0, "Aux 4"=999.0}}  # EPTxSettings_New_in
      }
    }
    "EPTxSettings" <- w46
    n14 = case shown="True" w9 {
      tunnel: [w100 w101] -> w58
      frame False {
        w100 = T1 {"Rotations"=0, "Cylinders"=0, "Primary"=[], "Aux 1"=[], "Aux 2"=[], "Aux 3"=[], "Aux 4"=[]}  # EPTxPatternSettings_0
      }
      frame True {
        w101 = T1 {"Rotations"=2, "Cylinders"=6, "Primary"=[{"Angle"=0.0, "State"=FALSE}, {"Angle"=3.0, "State"=TRUE}, {"Angle"=6.0, "State"=FALSE}, {"Angle"=9.0, "State"=TRUE}, {"Angle"=12.0, "State"=FALSE}, {"Angle"=15.0, "State"=TRUE}, {"Angle"=18.0, "State"=FALSE}, {"Angle"=21.0, "State"=TRUE}, {"Angle"=24.0, "State"=FALSE}, {"Angle"=27.0, "State"=TRUE}, {"Angle"=30.0, "State"=FALSE}, {"Angle"=33.0, "State"=TRUE}, {"Angle"=36.0, "State"=FALSE}, {"Angle"=39.0, "State"=TRUE}, {"Angle"=42.0, "State"=FALSE}, {"Angle"=45.0, "State"=TRUE}, {"Angle"=48.0, "State"=FALSE}, {"Angle"=51.0, "State"=TRUE}, {"Angle"=54.0, "State"=FALSE}, {"Angle"=57.0, "State"=TRUE}, {"Angle"=60.0, "State"=FALSE}, {"Angle"=63.0, "State"=TRUE}, {"Angle"=66.0, "State"=FALSE}, {"Angle"=69.0, "State"=TRUE}, {"Angle"=72.0, "State"=FALSE}, {"Angle"=75.0, "State"=TRUE}, {"Angle"=78.0, "State"=FALSE}, {"Angle"=81.0, "State"=TRUE}, {"Angle"=84.0, "State"=FALSE}, {"Angle"=87.0, "State"=TRUE}, {"Angle"=90.0, "State"=FALSE}, {"Angle"=93.0, "State"=TRUE}, {"Angle"=96.0, "State"=FALSE}, {"Angle"=99.0, "State"=TRUE}, {"Angle"=102.0, "State"=FALSE}, {"Angle"=105.0, "State"=TRUE}, {"Angle"=108.0, "State"=FALSE}, {"Angle"=111.0, "State"=TRUE}, {"Angle"=114.0, "State"=FALSE}, {"Angle"=117.0, "State"=TRUE}, {"Angle"=120.0, "State"=FALSE}, {"Angle"=123.0, "State"=TRUE}, {"Angle"=126.0, "State"=FALSE}, {"Angle"=129.0, "State"=TRUE}, {"Angle"=132.0, "State"=FALSE}, {"Angle"=135.0, "State"=TRUE}, {"Angle"=138.0, "State"=FALSE}, {"Angle"=141.0, "State"=TRUE}, {"Angle"=144.0, "State"=FALSE}, {"Angle"=147.0, "State"=TRUE}, {"Angle"=150.0, "State"=FALSE}, {"Angle"=153.0, "State"=TRUE}, {"Angle"=156.0, "State"=FALSE}, {"Angle"=159.0, "State"=TRUE}, {"Angle"=162.0, "State"=FALSE}, {"Angle"=165.0, "State"=TRUE}, {"Angle"=168.0, "State"=FALSE}, {"Angle"=171.0, "State"=TRUE}, {"Angle"=174.0, "State"=FALSE}, {"Angle"=177.0, "State"=TRUE}, {"Angle"=180.0, "State"=FALSE}, {"Angle"=183.0, "State"=TRUE}, {"Angle"=186.0, "State"=FALSE}, {"Angle"=189.0, "State"=TRUE}, {"Angle"=192.0, "State"=FALSE}, {"Angle"=195.0, "State"=TRUE}, {"Angle"=198.0, "State"=FALSE}, {"Angle"=201.0, "State"=TRUE}, {"Angle"=204.0, "State"=FALSE}, {"Angle"=207.0, "State"=TRUE}, {"Angle"=210.0, "State"=FALSE}, {"Angle"=213.0, "State"=TRUE}, {"Angle"=216.0, "State"=FALSE}, {"Angle"=219.0, "State"=TRUE}, {"Angle"=222.0, "State"=FALSE}, {"Angle"=225.0, "State"=TRUE}, {"Angle"=228.0, "State"=FALSE}, {"Angle"=231.0, "State"=TRUE}, {"Angle"=234.0, "State"=FALSE}, {"Angle"=237.0, "State"=TRUE}, {"Angle"=240.0, "State"=FALSE}, {"Angle"=243.0, "State"=TRUE}, {"Angle"=246.0, "State"=FALSE}, {"Angle"=249.0, "State"=TRUE}, {"Angle"=252.0, "State"=FALSE}, {"Angle"=255.0, "State"=TRUE}, {"Angle"=258.0, "State"=FALSE}, {"Angle"=261.0, "State"=TRUE}, {"Angle"=264.0, "State"=FALSE}, {"Angle"=267.0, "State"=TRUE}, {"Angle"=270.0, "State"=FALSE}, {"Angle"=273.0, "State"=TRUE}, {"Angle"=276.0, "State"=FALSE}, {"Angle"=279.0, "State"=TRUE}, {"Angle"=282.0, "State"=FALSE}, {"Angle"=285.0, "State"=TRUE}, {"Angle"=288.0, "State"=FALSE}, {"Angle"=291.0, "State"=TRUE}, {"Angle"=294.0, "State"=FALSE}, {"Angle"=297.0, "State"=TRUE}, {"Angle"=300.0, "State"=FALSE}, {"Angle"=303.0, "State"=TRUE}, {"Angle"=306.0, "State"=FALSE}, {"Angle"=309.0, "State"=TRUE}, {"Angle"=312.0, "State"=FALSE}, {"Angle"=315.0, "State"=TRUE}, {"Angle"=318.0, "State"=FALSE}, {"Angle"=321.0, "State"=TRUE}, {"Angle"=324.0, "State"=FALSE}, {"Angle"=327.0, "State"=TRUE}, {"Angle"=330.0, "State"=FALSE}, {"Angle"=333.0, "State"=TRUE}, {"Angle"=336.0, "State"=FALSE}, {"Angle"=339.0, "State"=TRUE}, {"Angle"=342.0, "State"=FALSE}, {"Angle"=345.0, "State"=TRUE}, {"Angle"=360.0, "State"=FALSE}, {"Angle"=363.0, "State"=TRUE}, {"Angle"=366.0, "State"=FALSE}, {"Angle"=369.0, "State"=TRUE}, {"Angle"=372.0, "State"=FALSE}, {"Angle"=375.0, "State"=TRUE}, {"Angle"=378.0, "State"=FALSE}, {"Angle"=381.0, "State"=TRUE}, {"Angle"=384.0, "State"=FALSE}, {"Angle"=387.0, "State"=TRUE}, {"Angle"=390.0, "State"=FALSE}, {"Angle"=393.0, "State"=TRUE}, {"Angle"=396.0, "State"=FALSE}, {"Angle"=399.0, "State"=TRUE}, {"Angle"=402.0, "State"=FALSE}, {"Angle"=405.0, "State"=TRUE}, {"Angle"=408.0, "State"=FALSE}, {"Angle"=411.0, "State"=TRUE}, {"Angle"=414.0, "State"=FALSE}, {"Angle"=417.0, "State"=TRUE}, {"Angle"=420.0, "State"=FALSE}, {"Angle"=423.0, "State"=TRUE}, {"Angle"=426.0, "State"=FALSE}, {"Angle"=429.0, "State"=TRUE}, {"Angle"=432.0, "State"=FALSE}, {"Angle"=435.0, "State"=TRUE}, {"Angle"=438.0, "State"=FALSE}, {"Angle"=441.0, "State"=TRUE}, {"Angle"=444.0, "State"=FALSE}, {"Angle"=447.0, "State"=TRUE}, {"Angle"=450.0, "State"=FALSE}, {"Angle"=453.0, "State"=TRUE}, {"Angle"=456.0, "State"=FALSE}, {"Angle"=459.0, "State"=TRUE}, {"Angle"=462.0, "State"=FALSE}, {"Angle"=465.0, "State"=TRUE}, {"Angle"=468.0, "State"=FALSE}, {"Angle"=471.0, "State"=TRUE}, {"Angle"=474.0, "State"=FALSE}, {"Angle"=477.0, "State"=TRUE}, {"Angle"=480.0, "State"=FALSE}, {"Angle"=483.0, "State"=TRUE}, {"Angle"=486.0, "State"=FALSE}, {"Angle"=489.0, "State"=TRUE}, {"Angle"=492.0, "State"=FALSE}, {"Angle"=495.0, "State"=TRUE}, {"Angle"=498.0, "State"=FALSE}, {"Angle"=501.0, "State"=TRUE}, {"Angle"=504.0, "State"=FALSE}, {"Angle"=507.0, "State"=TRUE}, {"Angle"=510.0, "State"=FALSE}, {"Angle"=513.0, "State"=TRUE}, {"Angle"=516.0, "State"=FALSE}, {"Angle"=519.0, "State"=TRUE}, {"Angle"=522.0, "State"=FALSE}, {"Angle"=525.0, "State"=TRUE}, {"Angle"=528.0, "State"=FALSE}, {"Angle"=531.0, "State"=TRUE}, {"Angle"=534.0, "State"=FALSE}, {"Angle"=537.0, "State"=TRUE}, {"Angle"=540.0, "State"=FALSE}, {"Angle"=543.0, "State"=TRUE}, {"Angle"=546.0, "State"=FALSE}, {"Angle"=549.0, "State"=TRUE}, {"Angle"=552.0, "State"=FALSE}, {"Angle"=555.0, "State"=TRUE}, {"Angle"=558.0, "State"=FALSE}, {"Angle"=561.0, "State"=TRUE}, {"Angle"=564.0, "State"=FALSE}, {"Angle"=567.0, "State"=TRUE}, {"Angle"=570.0, "State"=FALSE}, {"Angle"=573.0, "State"=TRUE}, {"Angle"=576.0, "State"=FALSE}, {"Angle"=579.0, "State"=TRUE}, {"Angle"=582.0, "State"=FALSE}, {"Angle"=585.0, "State"=TRUE}, {"Angle"=588.0, "State"=FALSE}, {"Angle"=591.0, "State"=TRUE}, {"Angle"=594.0, "State"=FALSE}, {"Angle"=597.0, "State"=TRUE}, {"Angle"=600.0, "State"=FALSE}, {"Angle"=603.0, "State"=TRUE}, {"Angle"=606.0, "State"=FALSE}, {"Angle"=609.0, "State"=TRUE}, {"Angle"=612.0, "State"=FALSE}, {"Angle"=615.0, "State"=TRUE}, {"Angle"=618.0, "State"=FALSE}, {"Angle"=621.0, "State"=TRUE}, {"Angle"=624.0, "State"=FALSE}, {"Angle"=627.0, "State"=TRUE}, {"Angle"=630.0, "State"=FALSE}, {"Angle"=633.0, "State"=TRUE}, {"Angle"=636.0, "State"=FALSE}, {"Angle"=639.0, "State"=TRUE}, {"Angle"=642.0, "State"=FALSE}, {"Angle"=645.0, "State"=TRUE}, {"Angle"=648.0, "State"=FALSE}, {"Angle"=651.0, "State"=TRUE}, {"Angle"=654.0, "State"=FALSE}, {"Angle"=657.0, "State"=TRUE}, {"Angle"=660.0, "State"=FALSE}, {"Angle"=663.0, "State"=TRUE}, {"Angle"=666.0, "State"=FALSE}, {"Angle"=669.0, "State"=TRUE}, {"Angle"=672.0, "State"=FALSE}, {"Angle"=675.0, "State"=TRUE}, {"Angle"=678.0, "State"=FALSE}, {"Angle"=681.0, "State"=TRUE}, {"Angle"=684.0, "State"=FALSE}, {"Angle"=687.0, "State"=TRUE}, {"Angle"=690.0, "State"=FALSE}, {"Angle"=693.0, "State"=TRUE}, {"Angle"=696.0, "State"=FALSE}, {"Angle"=699.0, "State"=TRUE}, {"Angle"=702.0, "State"=FALSE}, {"Angle"=705.0, "State"=TRUE}], "Aux 1"=[{"Angle"=12.0, "State"=TRUE}, {"Angle"=24.0, "State"=FALSE}, {"Angle"=48.0, "State"=TRUE}, {"Angle"=60.0, "State"=FALSE}, {"Angle"=132.0, "State"=TRUE}, {"Angle"=144.0, "State"=FALSE}, {"Angle"=198.0, "State"=TRUE}, {"Angle"=252.0, "State"=TRUE}, {"Angle"=264.0, "State"=FALSE}, {"Angle"=318.0, "State"=TRUE}, {"Angle"=372.0, "State"=TRUE}, {"Angle"=384.0, "State"=FALSE}, {"Angle"=438.0, "State"=TRUE}, {"Angle"=492.0, "State"=TRUE}, {"Angle"=504.0, "State"=FALSE}, {"Angle"=558.0, "State"=TRUE}, {"Angle"=612.0, "State"=TRUE}, {"Angle"=624.0, "State"=FALSE}, {"Angle"=678.0, "State"=TRUE}], "Aux 2"=[{"Angle"=12.0, "State"=TRUE}, {"Angle"=24.0, "State"=FALSE}, {"Angle"=48.0, "State"=TRUE}, {"Angle"=60.0, "State"=FALSE}, {"Angle"=132.0, "State"=TRUE}, {"Angle"=144.0, "State"=FALSE}, {"Angle"=198.0, "State"=TRUE}, {"Angle"=252.0, "State"=TRUE}, {"Angle"=264.0, "State"=FALSE}, {"Angle"=318.0, "State"=TRUE}, {"Angle"=372.0, "State"=TRUE}, {"Angle"=384.0, "State"=FALSE}, {"Angle"=438.0, "State"=TRUE}, {"Angle"=492.0, "State"=TRUE}, {"Angle"=504.0, "State"=FALSE}, {"Angle"=558.0, "State"=TRUE}, {"Angle"=612.0, "State"=TRUE}, {"Angle"=624.0, "State"=FALSE}, {"Angle"=678.0, "State"=TRUE}], "Aux 3"=[], "Aux 4"=[]}  # EPTxPatternSettings
      }
    }
    n15 = xnode "Read/Write Control"("FPGA VI Reference In"=w53, "error in"=w52) -> ("FPGA VI Reference Out"=w55:refnum<k20>, "error out"=w54:errorcluster, "EPTxSupervisor"=w87:T30)
    n16 = call <vilib>:"EPTx - Core Control.vi"("EPTxSupervisor"=w87, "Load"=w9, "EPTxSettings"=w46, "EPTxState"="EPTxState", "Frequency (40M) [Hz]"=w11, "Stall Speed (200) [RPM]"="Stall Speed [RPM]", "Filters (0)"="EPTxFilters", "History (63) [CAD]"="History [CAD]") -> ("EPTxConfig"=w90:T12, "EPTxControl"=w86:T31, "Max CAD"=w59:sgl, "EPTxData"=→"EPTxData":T19, "Loading"=→"Config Loading":bool)  [unwired: 3 in]
    "EPTxConfig" <- w90
    n17 = xnode "读取/写入控件"("FPGA VI Reference In"=w55, "error in"=w54, "EPTxConfig"=w90, "EPTxControl"=w86) -> ("FPGA VI Reference Out"=w50:refnum<k20>, "error out"=w51:errorcluster)
    n18 = Unbundle By Name("SimulatorConfig") -> ("Sim Speed [RPM]"=w10:sgl)
    n19 = call <vilib>:"Pattern Control.vi"("Load"=w9, "EPTxPatternSettings"=w58, "PatternConfig"="PatternConfig", "Frequency (40M) [Hz]"=w11) -> ("EPTxPatternConfig"=w77:T32, "Loading"=→"Pattern Loading":bool)  [unwired: 10 in]
    n20 = call <vilib>:"Simulation Control.vi"("SimulatorConfig"="SimulatorConfig", "Frequency (40M) [Hz]"=w11) -> ("EPTxSimulatorConfig"=w76:T11, "Loading"=→"Sim Loading":bool)  [unwired: 12 in]
    "EPTxSimulatorConfig" <- w76
    n21 = xnode "读取/写入控件"("FPGA VI Reference In"=w50, "error in"=w51, "EPTxPatternConfig"=w77, "EPTxSimulatorConfig"=w76) -> ("FPGA VI Reference Out"=w48:refnum<k20>, "error out"=w49:errorcluster, "EPTxDebug"=→"EPTxDebug":T34)
    n22 = call <vilib>:"Time2CAD.vi"("Time [ms]"="Injection_duration[ms]", "Speed (RPM)"=w10) -> ("CAD"=w17:sgl)
    n23 = Subtract(x=w37, y="Injection_DBTDC") -> (x-y=w36:sgl)
    n24 = Subtract(x=w43, y="Injection_DBTDC") -> (x-y=w39:sgl)
    n25 = Subtract(x=w27, y="Injection_DBTDC") -> (x-y=w26:sgl)
    n26 = Subtract(x=w22, y="Injection_DBTDC") -> (x-y=w21:sgl)
    n27 = Subtract(x=w33, y="Injection_DBTDC") -> (x-y=w31:sgl)
    n28 = Subtract(x=w18, y="Injection_DBTDC") -> (x-y=w15:sgl)
    n29 = call <vilib>:"AAP Config.vi"("Max CAD"=w59, "Cylinder TDC [Absolute CAD]"=w33, "EPTxAAPControl"="EPTxAAPControl_3str") -> ("EPTxAAPControl"=w68:T35)  [unwired: 8 in]
    n30 = call <vilib>:"AAP Config.vi"("Max CAD"=w59, "Cylinder TDC [Absolute CAD]"=w27, "EPTxAAPControl"="EPTxAAPControl_4str") -> ("EPTxAAPControl"=w67:T35)  [unwired: 8 in]
    n31 = call <vilib>:"AAP Config.vi"("Max CAD"=w59, "Cylinder TDC [Absolute CAD]"=w22, "EPTxAAPControl"="EPTxAAPControl_5str") -> ("EPTxAAPControl"=w66:T35)  [unwired: 8 in]
    n32 = call <vilib>:"AAP Config.vi"("Max CAD"=w59, "Cylinder TDC [Absolute CAD]"=w37, "EPTxAAPControl"="EPTxAAPControl_2str") -> ("EPTxAAPControl"=w69:T35)  [unwired: 8 in]
    n33 = call <vilib>:"AAP Config.vi"("Max CAD"=w59, "Cylinder TDC [Absolute CAD]"=w18, "EPTxAAPControl"="EPTxAAPControl_6str") -> ("EPTxAAPControl"=w65:T35)  [unwired: 8 in]
    n34 = call <vilib>:"AAP Config.vi"("Max CAD"=w59, "Cylinder TDC [Absolute CAD]"=w43, "EPTxAAPControl"="EPTxAAPControl_1str") -> ("EPTxAAPControl"=w73:T35)  [unwired: 8 in]
    n35 = Add(x=w39, y=w17) -> (x+y=w40:sgl)
    n36 = Add(x=w31, y=w17) -> (x+y=w30:sgl)
    n37 = Add(x=w36, y=w17) -> (x+y=w32:sgl)
    n38 = Add(x=w26, y=w17) -> (x+y=w25:sgl)
    n39 = Add(x=w21, y=w17) -> (x+y=w20:sgl)
    n40 = Add(x=w15, y=w17) -> (x+y=w14:sgl)
    n41 = Bundle By Name(cluster=w42, "Cylinder1_H_R [CAD]"=w39, "Cylinder1_H_F [CAD]"=w40) -> (w41:T29)
    n42 = Bundle By Name(cluster=w38, "Cylinder2_H_R [CAD]"=w36, "Cylinder2_H_F [CAD]"=w32) -> (w12:T28)
    n43 = Bundle By Name(cluster=w35, "Cylinder3_H_R [CAD]"=w31, "Cylinder3_H_F [CAD]"=w30) -> (w34:T27)
    n44 = Bundle By Name(cluster=w29, "Cylinder4_H_R [CAD]"=w26, "Cylinder4_H_F [CAD]"=w25) -> (w28:T26)
    n45 = Bundle By Name(cluster=w24, "Cylinder5_H_R [CAD]"=w21, "Cylinder5_H_F [CAD]"=w20) -> (w23:T25)
    n46 = Bundle By Name(cluster=w16, "Cylinder6_H_R [CAD]"=w15, "Cylinder6_H_F [CAD]"=w14) -> (w13:T24)
    n47 = xnode "读取/写入控件"("FPGA VI Reference In"=w48, "error in"=w49, "AAPControl_1str"=w73, "AAPControl_2str"=w69, "AAPControl_3str"=w68, "AAPControl_4str"=w67, "AAPControl_5str"=w66, "AAPControl_6str"=w65, "CylinderSig_1"=w41, "CylinderSig_2"=w12, "CylinderSig_3"=w34, "CylinderSig_4"=w28, "CylinderSig_5"=w23, "CylinderSig_6"=w13) -> ("FPGA VI Reference Out"=w80:refnum<k20>, "error out"=w79:errorcluster, "Loop"=→"Loop":u32)
    n48 = node-c288(w79) -> ()  [unwired: 1 out]
  }
  n49 = node-c288(w6) -> (w4:errorcluster)
  n50 = xnode "Close FPGA VI Reference"("FPGA VI Reference In"=w5, "error in"=w4) -> ("error out"=→"error out":errorcluster)
